vi "Axis Camera Config UI.vi"() -> ()   [LabVIEW 2017]
panel:
  out "Image":T1(plugin-control)
  in  "Done":bool
  in  "Black Level Correction":dbl
  in  "Sharpness":i32 min=-2 max=2
  in  "Color Level":i32 min=0 max=100
  in  "Brightness":i32 min=0 max=100
  in  "Exposure Priority":T2(ring)
  in  "Exposure":T3(ring)
  in  "White Balance":T4(ring)
  in  "IP Address":string="192.168.0.90"
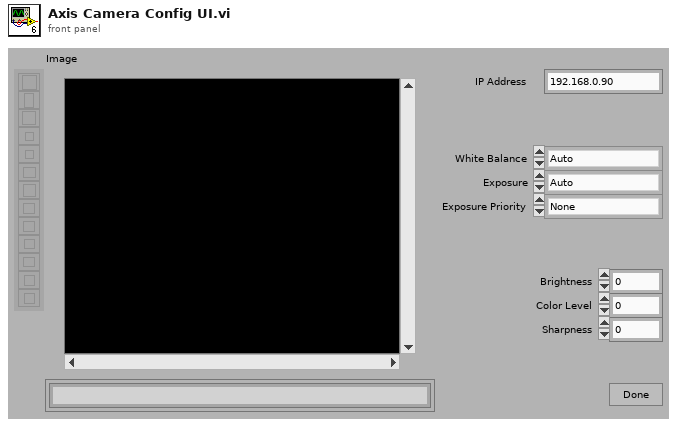
[diagram p1: front panel]
types:
  T1 = typedef "IMAQ Image.ctl" = refnum<image>
  T2 = enum16{"None", "Prioritize framerate", "Prioritizeimage quality"}
  T3 = enum16{"Auto", "Flicker-free 50 Hz", "Flicker-free 60 Hz", "Hold current"}
  T4 = enum16{"Auto", "Fixed Indoor", "Fixed Outdoor 1", "Fixed Outdoor 2", "Fixed Fluorescent 1", "Fixed Fluorescent 2", "Hold current"}
  T5 = typedef "Image Type" = u32
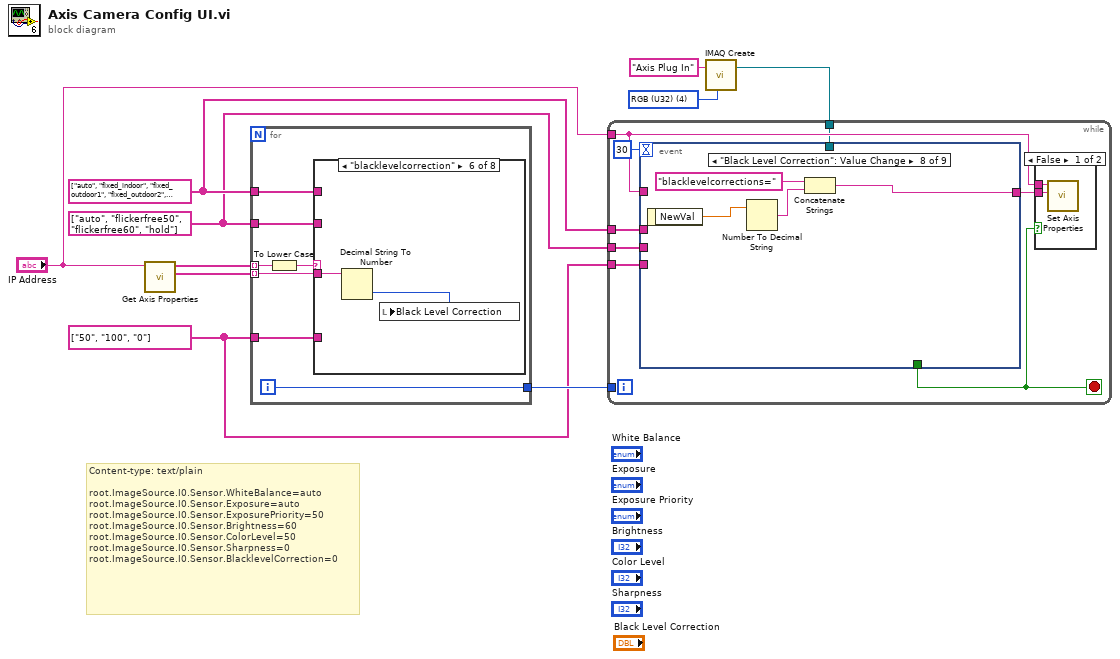
[diagram p0: block diagram]
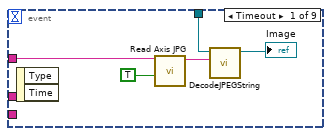
[diagram p3: hidden frame]
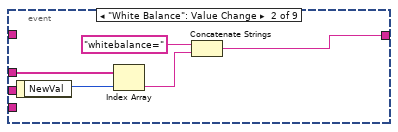
[diagram p4: hidden frame]
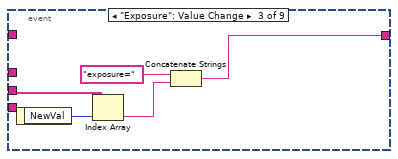
[diagram p5: hidden frame]
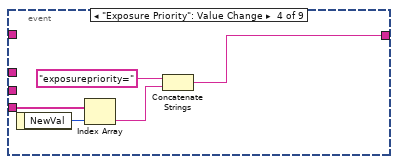
[diagram p6: hidden frame]
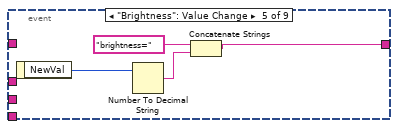
[diagram p7: hidden frame]
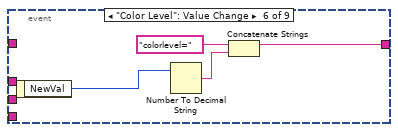
[diagram p8: hidden frame]
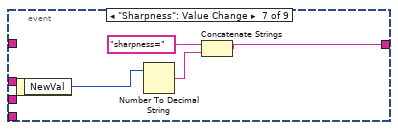
[diagram p9: hidden frame]
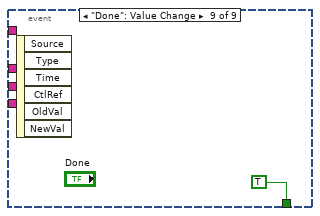
[diagram p10: hidden frame]
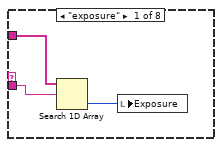
[diagram p11: hidden frame]
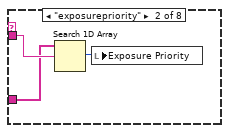
[diagram p12: hidden frame]
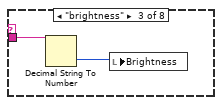
[diagram p13: hidden frame]
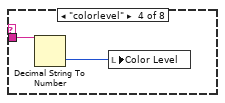
[diagram p14: hidden frame]
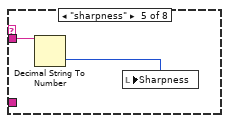
[diagram p15: hidden frame]
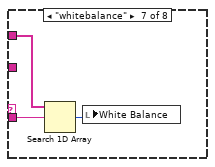
[diagram p16: hidden frame]
diagram:
  w2 = T5 4 items=["Grayscale (U8)", "Grayscale (I16)", "Grayscale (SGL)", "Complex (CSG)", "RGB (U32)", "HSL (U32)", "RGB (U64)"] ("Image Type")
  w4 = string[] ["50", "100", "0"]
  w5 = string[] ["auto", "flickerfree50", "flickerfree60", "hold"]
  w6 = string[] ["auto", "fixed_indoor", "fixed_outdoor1", "fixed_outdoor2", "fixed_fluor1", "fixed_fluor2", "hold", "fixed_fluor", "fixed_outdoor"]
  # "Content-type: text/plain\n\nroot.ImageSource.I0.Sensor.WhiteBalance=auto\nroot.ImageSource.I0.Sensor.Exposure=auto\nroot.ImageSource.I0.Sensor.ExposurePriority=50\nroot.ImageSource.I0.Sensor.Brightness=60\nroot.ImageSource.I0.Sensor.ColorLevel=50\nroot.ImageSource.I0.Sensor.Sharpness=0\nroot.ImageSource.I0.Sensor.BlacklevelCorrection=0"
  n1 = call <vilib>:"Get Axis Properties.vi"("address"="IP Address") -> ("Values"=w9:string[], "Prop Names"=w10:string[])  [unwired: 8 in, 1 out]
  n2 = for {
    tunnel: w10 -> [w17] mode=indexing
    tunnel: w9 -> [w15] mode=indexing
    tunnel: w6 -> [w14]
    tunnel: w5 -> [w13]
    tunnel: w4 -> [w12]
    tunnel: [w11] -> w8
    i -> [w11]
    n3 = To Lower Case(string=w17) -> (all lower case string=w16:string)
    n4 = case shown="\"blacklevelcorrection\"" w16 {
      tunnel: w15 -> [w19 w22 w25 w27 w29 w31 w32 _]
      tunnel: w14 -> [_ _ _ _ _ _ w33 _]
      tunnel: w13 -> [w20 _ _ _ _ _ _ _]
      tunnel: w12 -> [_ w21 _ _ _ _ _ _]
      frame "exposure" {
        n5 = Search 1D Array(1D array=w20, element=w19) -> (index of element=w18:i32)  [unwired: 1 in]
        n6 = local write "Exposure"(w18) -> ()
      }
      frame "exposurepriority" {
        n7 = Search 1D Array(1D array=w21, element=w22) -> (index of element=w23:i32)  [unwired: 1 in]
        n8 = local write "Exposure Priority"(w23) -> ()
      }
      frame "brightness" {
        n9 = Decimal String To Number(string=w25) -> (number=w24:i32)  [unwired: 2 in, 1 out]
        n10 = local write "Brightness"(w24) -> ()
      }
      frame "colorlevel" {
        n11 = Decimal String To Number(string=w27) -> (number=w26:i32)  [unwired: 2 in, 1 out]
        n12 = local write "Color Level"(w26) -> ()
      }
      frame "sharpness" {
        n13 = Decimal String To Number(string=w29) -> (number=w28:i32)  [unwired: 2 in, 1 out]
        n14 = local write "Sharpness"(w28) -> ()
      }
      frame "blacklevelcorrection" {
        n15 = Decimal String To Number(string=w31) -> (number=w30:i32)  [unwired: 2 in, 1 out]
        n16 = local write "Black Level Correction"(w30) -> ()
      }
      frame "whitebalance" {
        n17 = Search 1D Array(1D array=w33, element=w32) -> (index of element=w34:i32)  [unwired: 1 in]
        n18 = local write "White Balance"(w34) -> ()
      }
      frame Default {
      }
    }
  }
  n19 = call "IMAQ Create"("Image Name"="Axis Plug In", "Image Type"=w2) -> ("New Image"=w1:T1)  [unwired: 3 in, 1 out]
  n20 = while {
    tunnel: w8 -> [_]
    tunnel: "IP Address" -> [w37]
    tunnel: w6 -> [w40]
    tunnel: w5 -> [w39]
    tunnel: w4 -> [w38]
    tunnel: w1 -> [w36]
    stop <- w41 stop-if-true
    n21 = event shown="[7] \"Black Level Correction\": Value Change" {
      selector: _ -> [_ _ _ _ _ _ _ _ _]
      dyn-events: _ -> [_ _ _ _ _ _ _ _ _]
      timeout: 30 -> [_ _ _ _ _ _ _ _ _]
      tunnel: [_ _ _ _ _ _ _ _ TRUE] -> w41
      tunnel: [_ w50 w55 w60 w65 w70 w74 w78 _] -> w42
      tunnel: w40 -> [_ w53 _ _ _ _ _ _ _]
      tunnel: w39 -> [_ _ w56 _ _ _ _ _ _]
      tunnel: w38 -> [_ _ _ w61 _ _ _ _ _]
      tunnel: w37 -> [w49 _ _ _ _ _ _ _ _]
      tunnel: w36 -> [w46 _ _ _ _ _ _ _ _]
      event Timeout {
        n22 = event-data() -> ()  [unwired: 1 in, 2 out]
        n23 = call <vilib>:"Read Axis JPG.vi"("CGI?"=TRUE, "address"=w49) -> ("Raw Image Data"=w47:string)  [unwired: 8 in, 1 out]
        n24 = call <vilib>:"DecodeJPEGString.vi"("Compressed Image"=w47, "Image In"=w46) -> ("Image Out"=→"Image":T1)  [unwired: 4 in, 1 out]
      }
      event "White Balance": Value Change {
        n25 = event-data() -> ("NewVal"=w52:T4)  [unwired: 1 in]
        n26 = Index Array(array=w53, index=w52) -> (element=w51:string)
        n27 = Concatenate Strings("whitebalance=" ("Prop String"), w51) -> (w50:string)
      }
      event "Exposure": Value Change {
        n28 = event-data() -> ("NewVal"=w57:T3)  [unwired: 1 in]
        n29 = Index Array(array=w56, index=w57) -> (element=w58:string)
        n30 = Concatenate Strings("exposure=" ("Prop String"), w58) -> (w55:string)
      }
      event "Exposure Priority": Value Change {
        n31 = event-data() -> ("NewVal"=w62:T2)  [unwired: 1 in]
        n32 = Index Array(array=w61, index=w62) -> (element=w63:string)
        n33 = Concatenate Strings("exposurepriority=" ("Prop String"), w63) -> (w60:string)
      }
      event "Brightness": Value Change {
        n34 = event-data() -> ("NewVal"=w68:i32)  [unwired: 1 in]
        n35 = Number To Decimal String(number=w68) -> (decimal integer string=w66:string)  [unwired: 1 in]
        n36 = Concatenate Strings("brightness=" ("Prop String"), w66) -> (w65:string)
      }
      event "Color Level": Value Change {
        n37 = event-data() -> ("NewVal"=w69:i32)  [unwired: 1 in]
        n38 = Number To Decimal String(number=w69) -> (decimal integer string=w71:string)  [unwired: 1 in]
        n39 = Concatenate Strings("colorlevel=" ("Prop String"), w71) -> (w70:string)
      }
      event "Sharpness": Value Change {
        n40 = event-data() -> ("NewVal"=w73:i32)  [unwired: 1 in]
        n41 = Number To Decimal String(number=w73) -> (decimal integer string=w75:string)  [unwired: 1 in]
        n42 = Concatenate Strings("sharpness=" ("Prop String"), w75) -> (w74:string)
      }
      event "Black Level Correction": Value Change {
        n43 = event-data() -> ("NewVal"=w77:dbl)  [unwired: 1 in]
        n44 = Number To Decimal String(number=w77) -> (decimal integer string=w79:string)  [unwired: 1 in]
        n45 = Concatenate Strings("blacklevelcorrections=" ("Prop String"), w79) -> (w78:string)
      }
      event "Done": Value Change {
        n46 = event-data() -> ()  [unwired: 1 in, 6 out]
      }
    }
    n47 = case shown="False" w41 {
      tunnel: w37 -> [w44 _]
      tunnel: w42 -> [w43 _]
      frame False {
        n48 = call <vilib>:"Set Axis Properties.vi"("Prop String"=w43, "address"=w44) -> ()  [unwired: 9 in, 1 out]
      }
      frame True {
      }
    }
  }
